vi "Configure IQ vs Slot Measurement Trigger Mode.vi"(8 "error in (no error)":errorcluster, 9 "Mode (Once)":i32(ring) items=["Once", "Preselect"], 10 "Instance (1)":i32=1, 11 "VISA resource name":refnum<visa-resource-name>) -> (0 "error out":errorcluster, 3 "VISA resource name out":refnum<visa-resource-name>)   [LabVIEW 2015, in "Rohde&Schwarz CMXP GPRF.lvlib"]
doc: "Selects the measurement sequence that is triggered by each single trigger event. This setting is not valid for \"Free Run\" measurements.\n\nAttribute:\nRSCMXPGPRF_ATTR_IQ_VS_SLOT_MEASUREMENT_TRIGGER_MODE\n\nRemote-control command:\nTRIGger:GPRF:MEAS<i>:IQVSlot:MODE"
uses:
  <instrlib>/Rohde&Schwarz CMXP GPRF/Rohde&Schwarz CMXP GPRF.lvlib
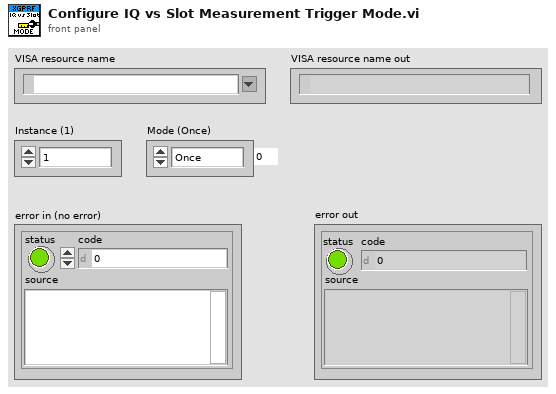
[diagram p1: front panel]
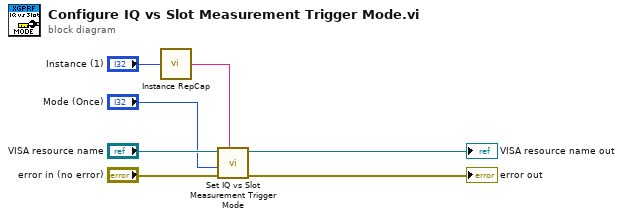
[diagram p0: block diagram]
diagram:
  n1 = call <instrlib>:"Instance RepCap.vi"("instance  in"="Instance (1)") -> ("instance out"=w6:string)
  n2 = call "Set IQ vs Slot Measurement Trigger Mode"("Repeated Capabilities"=w6, "error in (no error)"="error in (no error)", "IQ vs Slot Measurement Trigger Mode (0 - Once)"="Mode (Once)", "instrument handle"="VISA resource name") -> ("error out"=→"error out":errorcluster, "instrument handle out"=→"VISA resource name out":refnum<visa-resource-name>)  [unwired: 6 in]
